vi "Demo_Main.vi"() -> ()   [LabVIEW 2016]
uses:
  ControlCAN/ControlCAN.llb/DevType.ctl
  ControlCAN/ControlCAN.llb/CAN Channel.ctl
  ControlCAN/ControlCAN.llb/InitFlag.ctl
  ControlCAN/ControlCAN.llb/Mode.ctl
  ControlCAN/ControlCAN.llb/Fliter.ctl
  ControlCAN/ControlCAN.llb/VCI_CAN_OBJ.ctl
  ControlCAN/ControlCAN.llb/VCI_INIT_CONFIG.ctl
  ControlCAN/ControlCAN.llb/Return Val.ctl
  ControlCAN/ControlCAN.lvlib
panel:
  in  "元素 8":u8 format="%x"
  in  "元素 7":u8 format="%x"
  in  "元素 6":u8 format="%x"
  in  "元素 5":u8 format="%x"
  in  "元素 4":u8 format="%x"
  in  "元素 3":u8 format="%x"
  in  "元素 2":u8 format="%x"
  in  "元素":u8 format="%x"
  in  "单选按钮 3":enum32{"未选择", "逆转", "顺转", "输出锁定"}(radio)=enum."输出锁定"
  in  "ID_VCU_MCU_1 2":u32=150013185 format="0x%x"
  out "vcu1 2":u32[](array[numeric]) format="%x"
  out "vcu1":u32[](array[numeric]) format="%x"
  out "vcu2":u32[](array[numeric]) format="%x"
  out "控制器温度":i16
  in  "list":i32(listbox)
  out "vcu3":u32[](array[numeric]) format="%x"
  in  "Data":string="01 00"
  in  "Format":u8(ring)=1 items=["标准帧", "扩展帧"]
  in  "Type":u8(ring) items=["数据帧", "远程帧"]
  in  "ID":u32 format="0x%x"
  in  "Send":bool
  out "Open":bool
  in  "Open 2":bool
  in  "Close":bool
  in  "kBaudRate":u8(ring)=10 caption="波特率" items=["5k bps"=1, "10k bps"=2, "20k bps"=3, "40k bps"=4, "50k bps"=5, "80k bps"=6, "100k bps"=7, "125k bps"=8, "200k bps"=9, "250k bps"=10, "400k bps"=11, "500k bps"=12, "666k bps"=13, "800k bps"=14, "1000k bps"=15, "33.33k bps"=16, "66.66k bps"=17, "83.33k bps"=18]
  in  "Channel":T1 caption="CAN通道" items=["通道1", "通道2"]
  in  "DevType":T2=3 caption="设备类型" items=["USB-CAN"=2, "USB-CAN2"=3]
  in  "RcvEnable":bool=TRUE
  in  "InitFlag":T3=1 caption="初始化参数" items=["使用Flash参数", "使用界面设置参数"]
  out "选项卡控件":enum32{"VCU控制", "CAN基本操作"}(tab)
  in  "驱动/制动":enum32{"未选择", "N", "L"}(radio)=enum."N"
  in  "车辆动力":enum32{"未选择", "N", "L", "R"}(radio)=enum."R"
  in  "车辆状态":enum32{"未选择", "N", "L", "R"}(radio)=enum."L"
  in  "充电状态":T4(radio)=enum."单选选项1 4"
  in  "状态信息1":T4(radio)=enum."空"
  in  "ID_VCU_MCU_2 2":u32=150078721 format="0x%x"
  in  "ID_VCU_MCU_1":u32=150013185 format="0x%x"
  in  "单选按钮":enum32{"未选择", "运行", "停止"}(radio)=enum."停止"
  in  "单选按钮 2":enum32{"未选择", "牵引", "制动"}(radio)=enum."制动"
  in  "ID_VCU_MCU_33":u32=150930689 format="0x%x"
  in  "状态信息2":T5(radio)
  in  "报警信息":enum32{"未选择", "N", "L", "R", "R 2"}(radio)
  in  "制动":dbl(knob) scale=0.0..5.0
  in  "油门":dbl(knob) scale=0.0..5.0
  out "油门":dbl
  out "转矩":dbl
  out "转速":dbl
  out "单选按钮 4":enum32{"未选择", "逆转", "顺转", "输出锁定"}(radio)
  out "单选按钮 5":enum32{"未选择", "牵引", "制动"}(radio)
  out "单选按钮 6":enum32{"未选择", "运行", "停止"}(radio)
  out "布尔数组":bool[](array[boolean])
  out "母线电压":u16
  out "电机相电流":dbl
  out "电机实际功率":dbl
  out "电机温度":i16
  in  "Clear":bool
  in  "Mode":T6 caption="工作模式" items=["正常工作", "仅侦听模式", "自测模式（环回）"]
  in  "Fliter":T7=1 items=["接收所有类型"=1, "只接收标准帧"=2, "只接收扩展帧"=3]
  in  "AccMask":u32=4294967295 caption="接收屏蔽码" format="%08x"
  in  "AccCode":u32 caption="接收过滤码" format="%08x"
  out "SendCnt":u32 caption="发送统计"
  out "RecvCnt":u32 caption="接收统计"
  # "位置传感器故障"
  # "过流"
  # "控制器过温"
  # "电机过温"
  # "欠压报警"
  # "过压报警"
  # "通讯故障"
  # "控制器高温"
  # "短路保护"
  # "严重欠压"
  # "超过峰值功率"
  # "超过最高限速"
  # "VCU故障"
  # "跛行状态"
  # "堵转保护"
  # "致命故障"
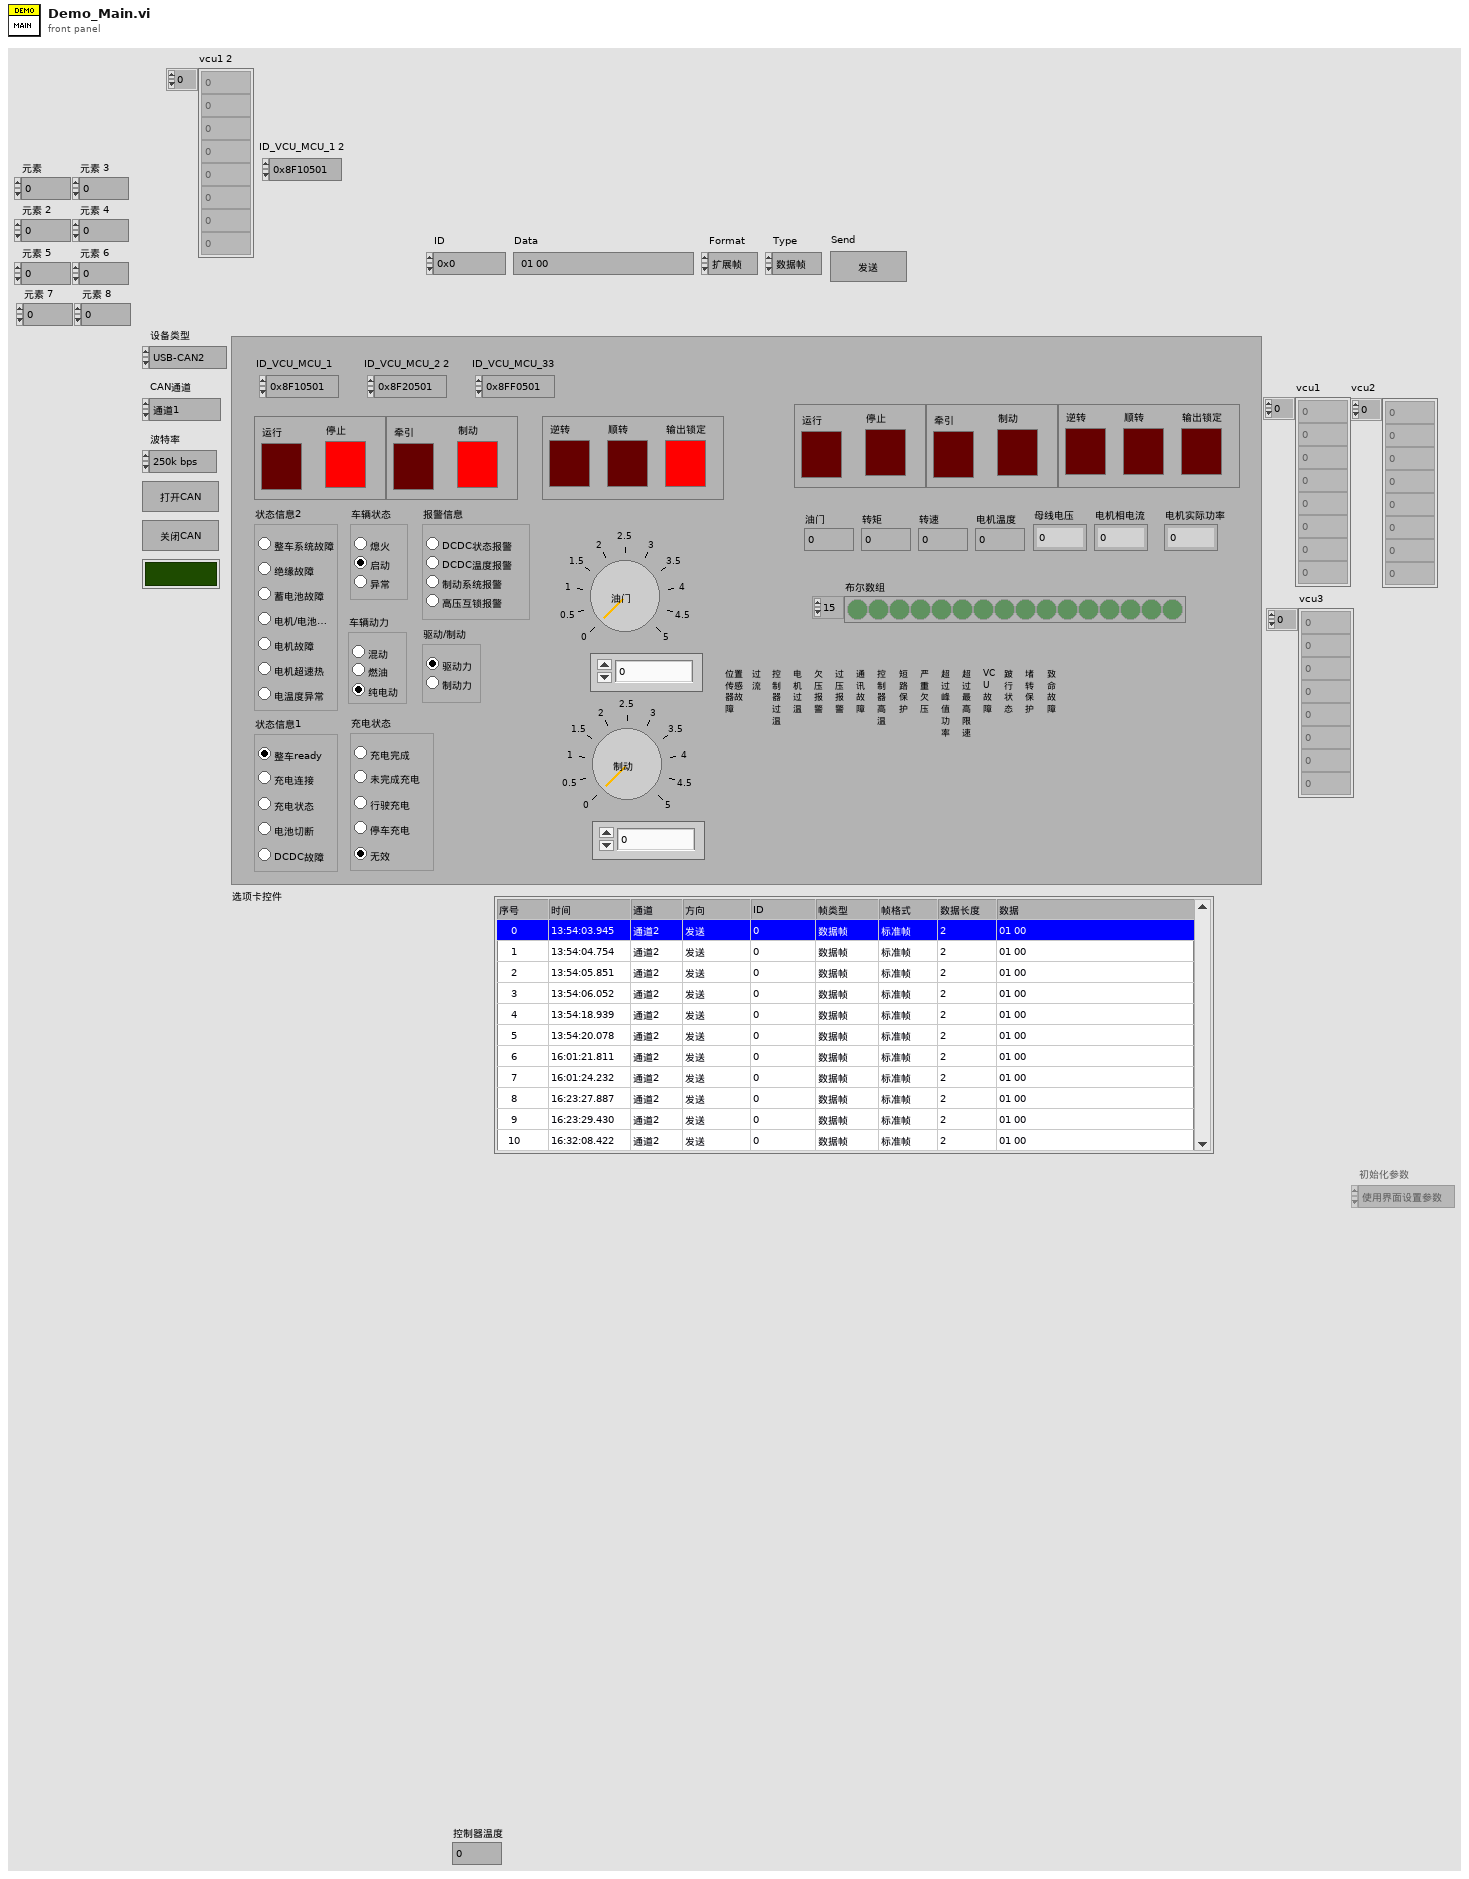
[diagram p1: front panel]
types:
  T1 = typedef "ControlCAN.lvlib/CAN Channel.ctl" = u32
  T2 = typedef "ControlCAN.lvlib/DevType.ctl" = u32
  T3 = typedef "ControlCAN.lvlib/InitFlag.ctl" = u32
  T4 = enum32{"未选择", "空", "速度控制", "转矩控制", "主动放电", "单选选项1 4"}
  T5 = enum32{"未选择", "空", "速度控制", "转矩控制", "主动放电", "单选选项1 4", "主动放电 2", "单选选项1 5"}
  T6 = typedef "ControlCAN.lvlib/Mode.ctl" = u8
  T7 = typedef "ControlCAN.lvlib/Fliter.ctl" = u8
  T8 = typedef "ControlCAN.lvlib/VCI_CAN_OBJ.ctl" = cluster{"ID":u32, "TimeStamp":u32, "TimeFlag":u8, "SendType":u8, "RemoteFlag":u8, "ExternFlag":u8, "DataLen":u8, "Data":u8[], "Reserved":u8[]}
  T9 = cluster{"Type":enum16{"接收", "发送"}, "Channel":T1, "Time":timestamp, "VCI_CAN_OBJ":T8}[]
  T10 = cluster{"Type":enum16{"接收", "发送"}, "Channel":T1, "Time":timestamp, "VCI_CAN_OBJ":T8}
  T11 = typedef "ControlCAN.lvlib/VCI_INIT_CONFIG.ctl" = cluster{"AccCode":u32, "AccMask":u32, "InitFlag":T3, "Fliter":T7, "Timing0":u8, "Timing1":u8, "Mode":T6}
  T12 = cluster{"DevType":T2, "DevIndex":u32, "CanIndex":T1, "VCI_INIT_CONFIG":T11}
  T13 = typedef "ControlCAN.lvlib/Return Val.ctl" = i32
  T14 = enum32{"invalid app kind", "Development System", "Run Time System", "Student Edition", "Embedded LabVIEW", "Evaluation", "Custom"}
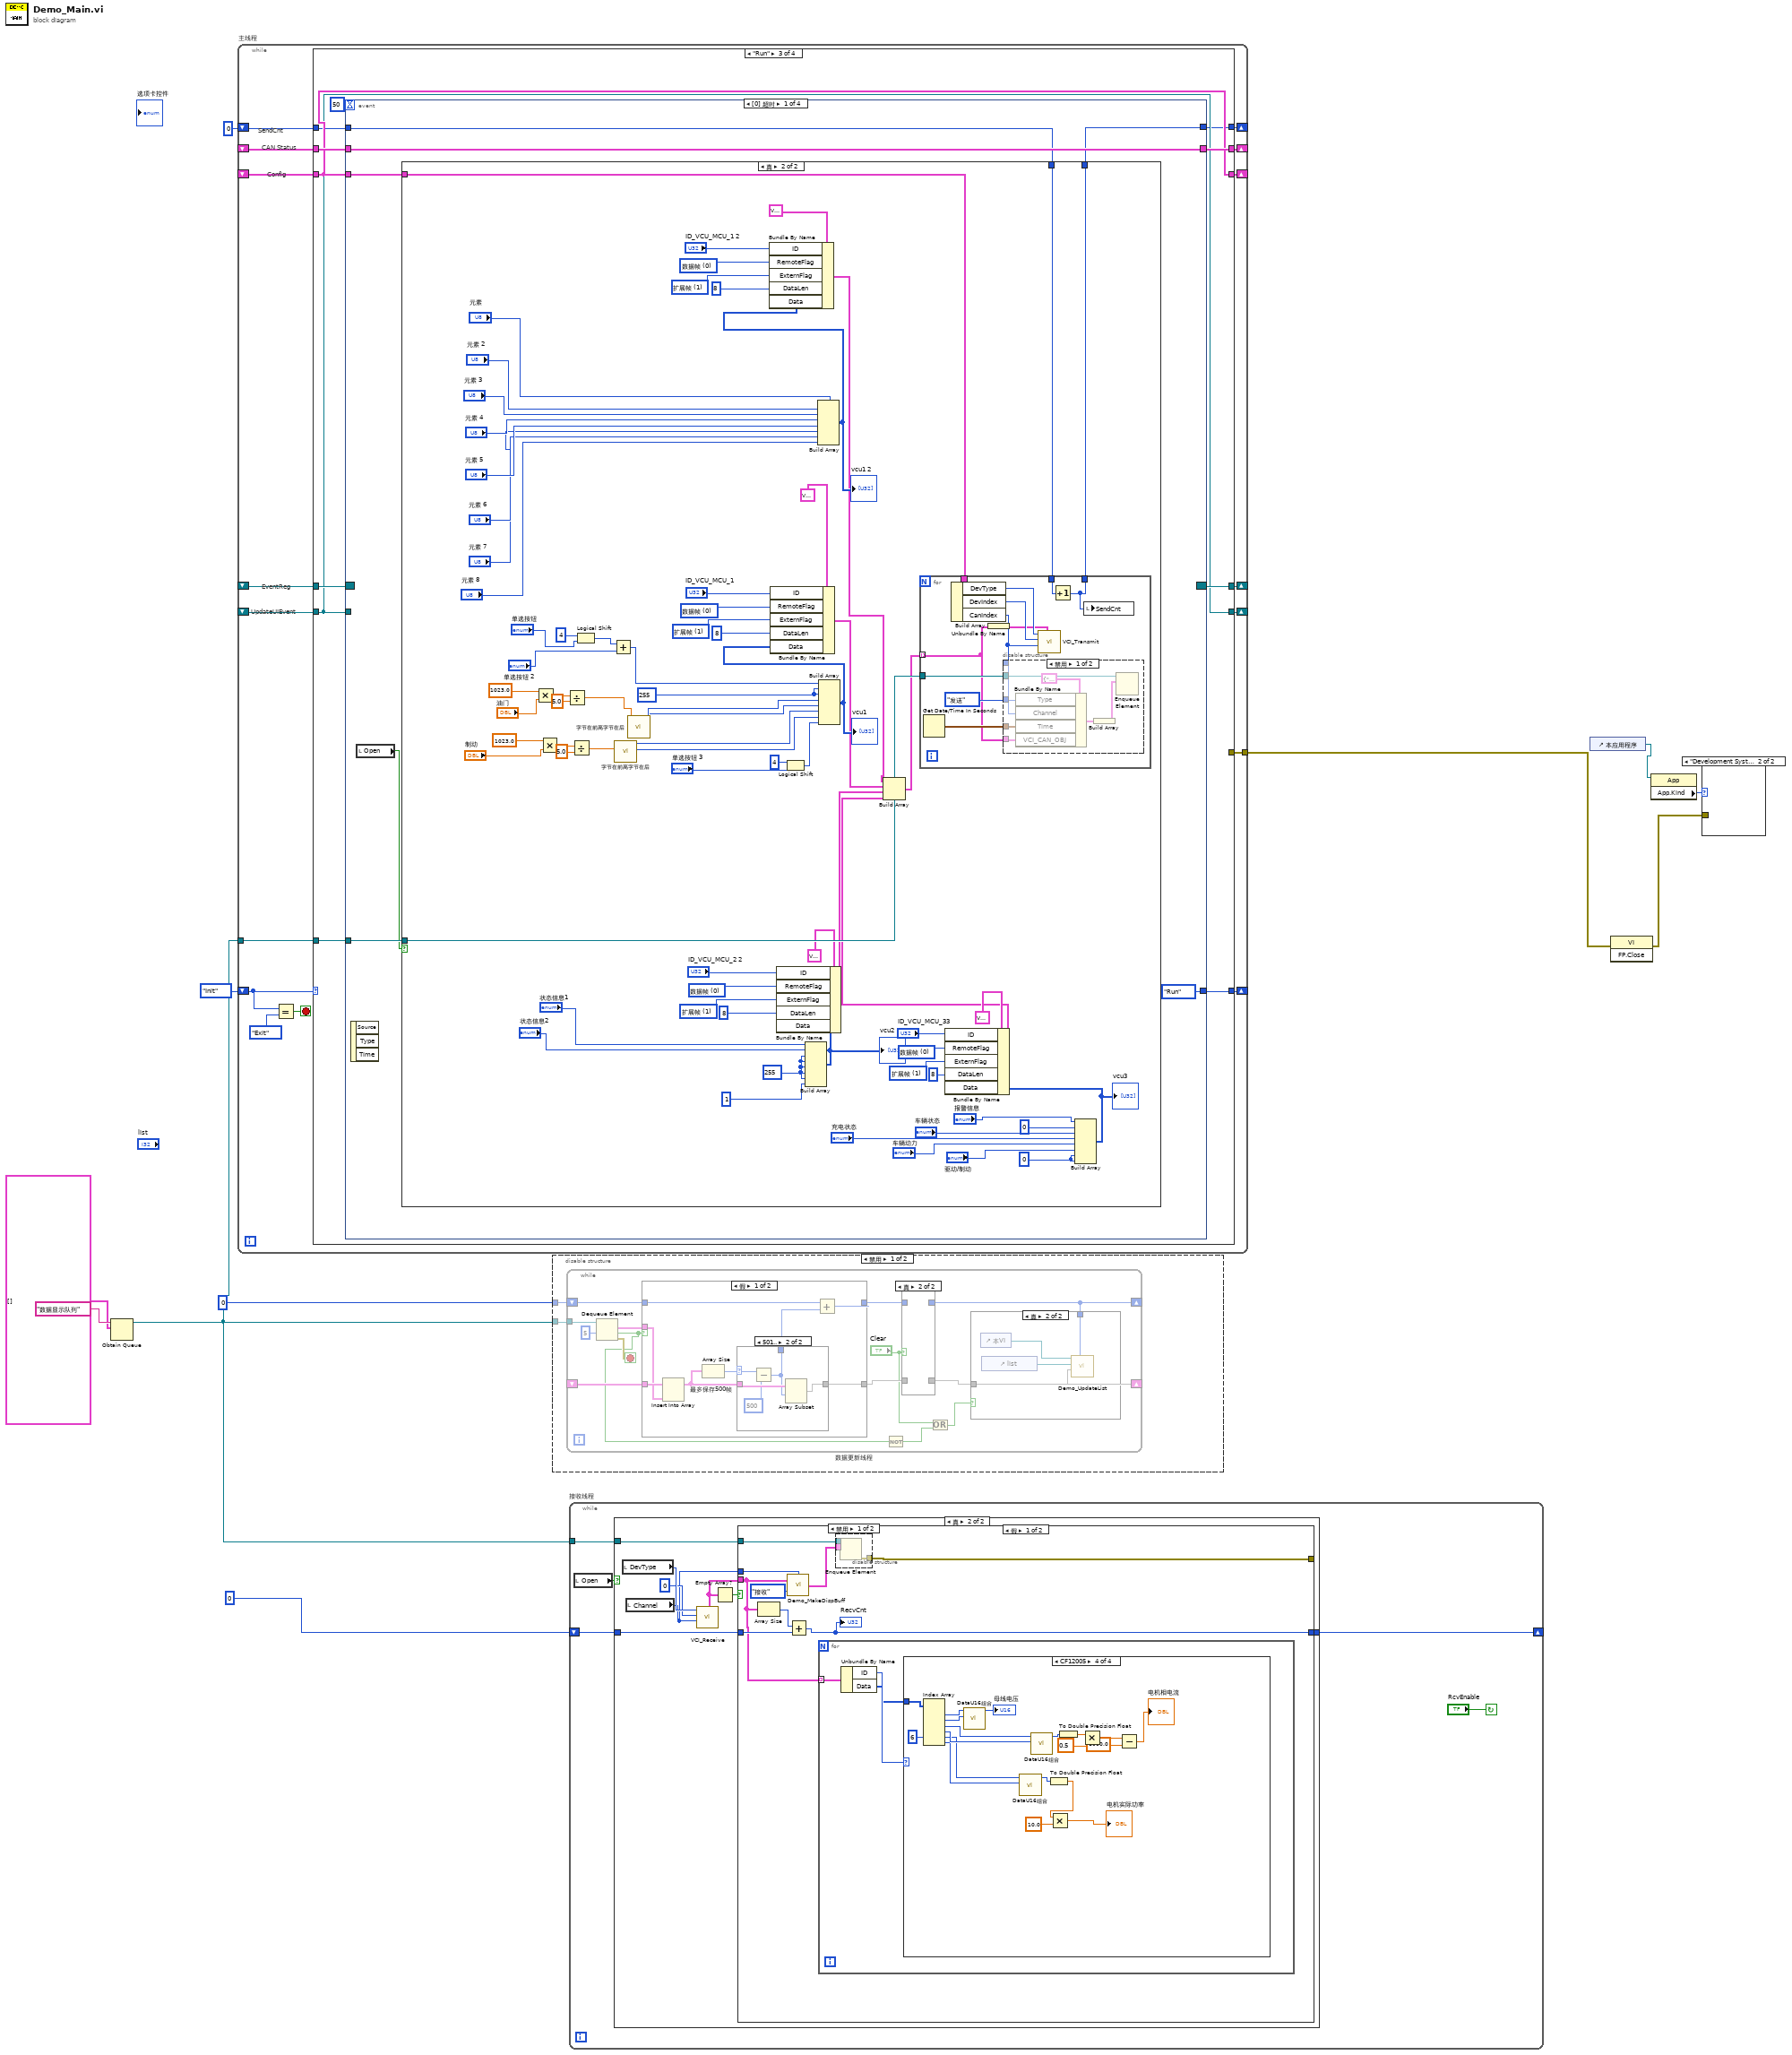
[diagram p0: block diagram]
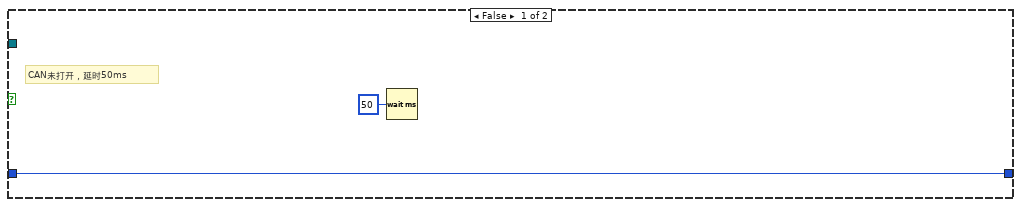
[diagram p7: hidden frame]
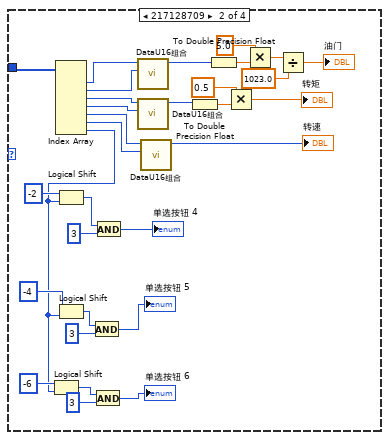
[diagram p10: hidden frame]
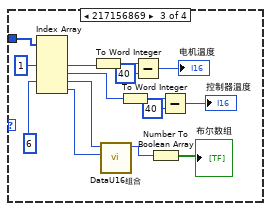
[diagram p11: hidden frame]
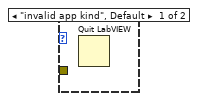
[diagram p13: hidden frame]
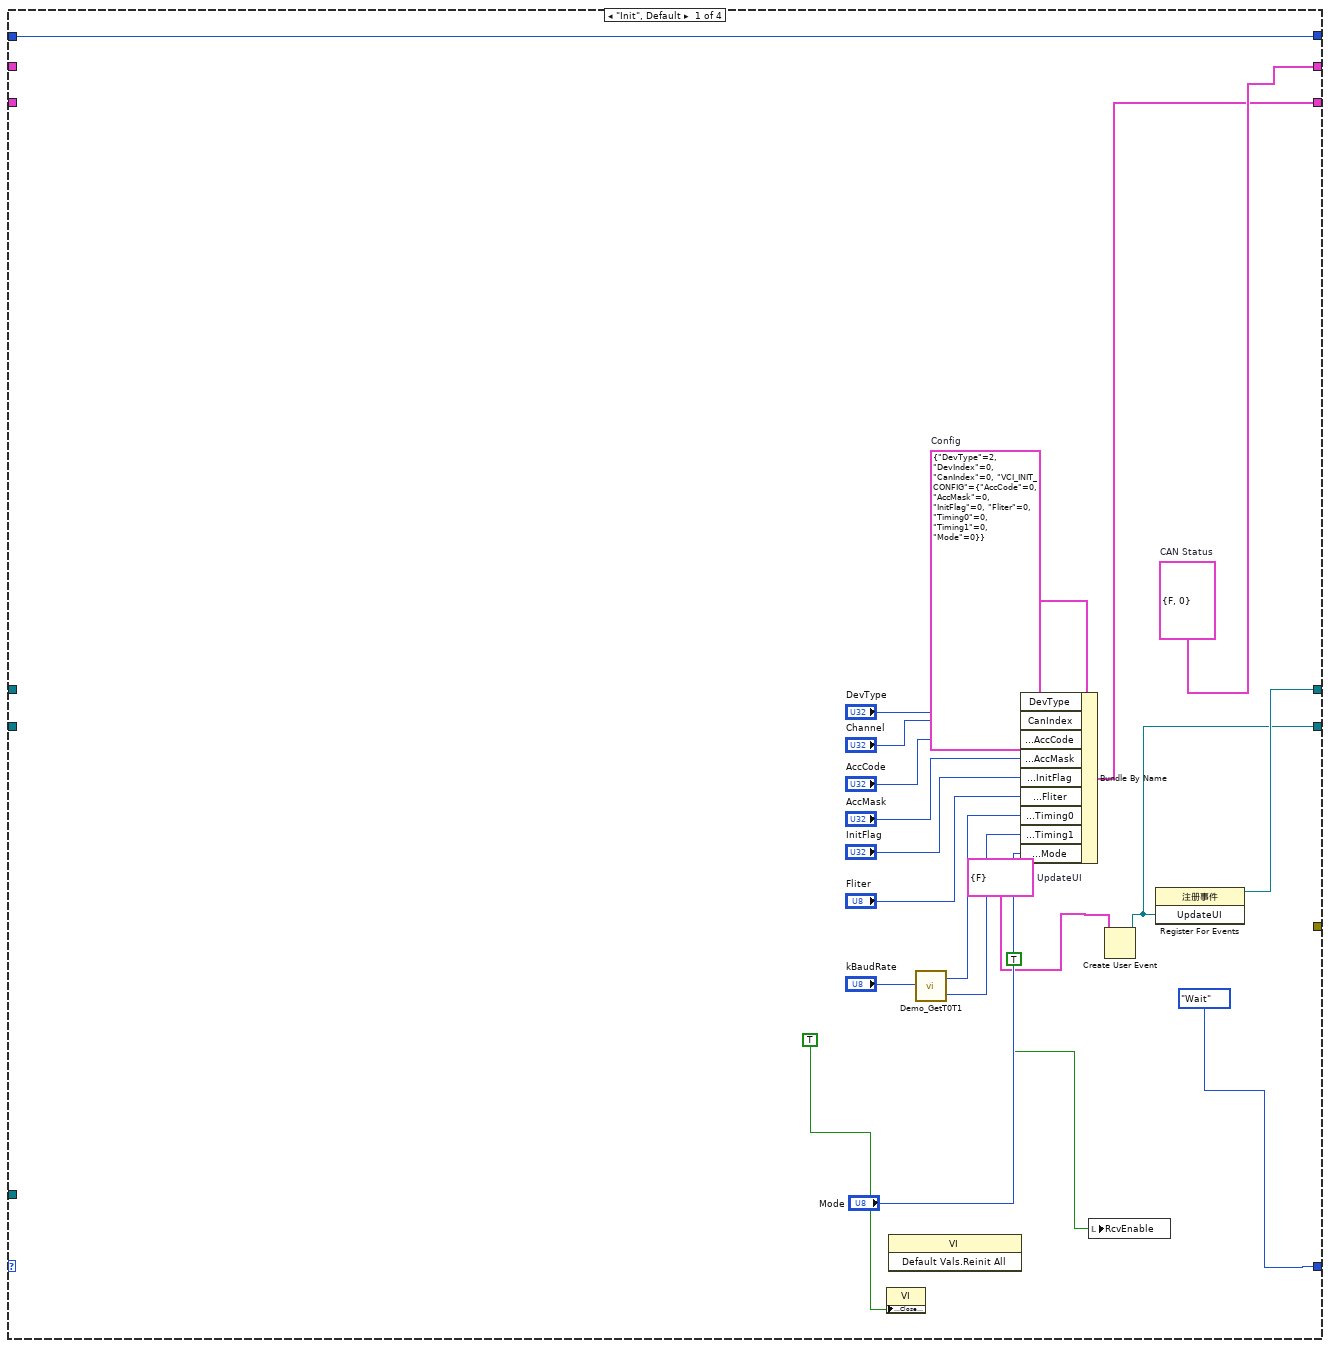
[diagram p14: hidden frame]
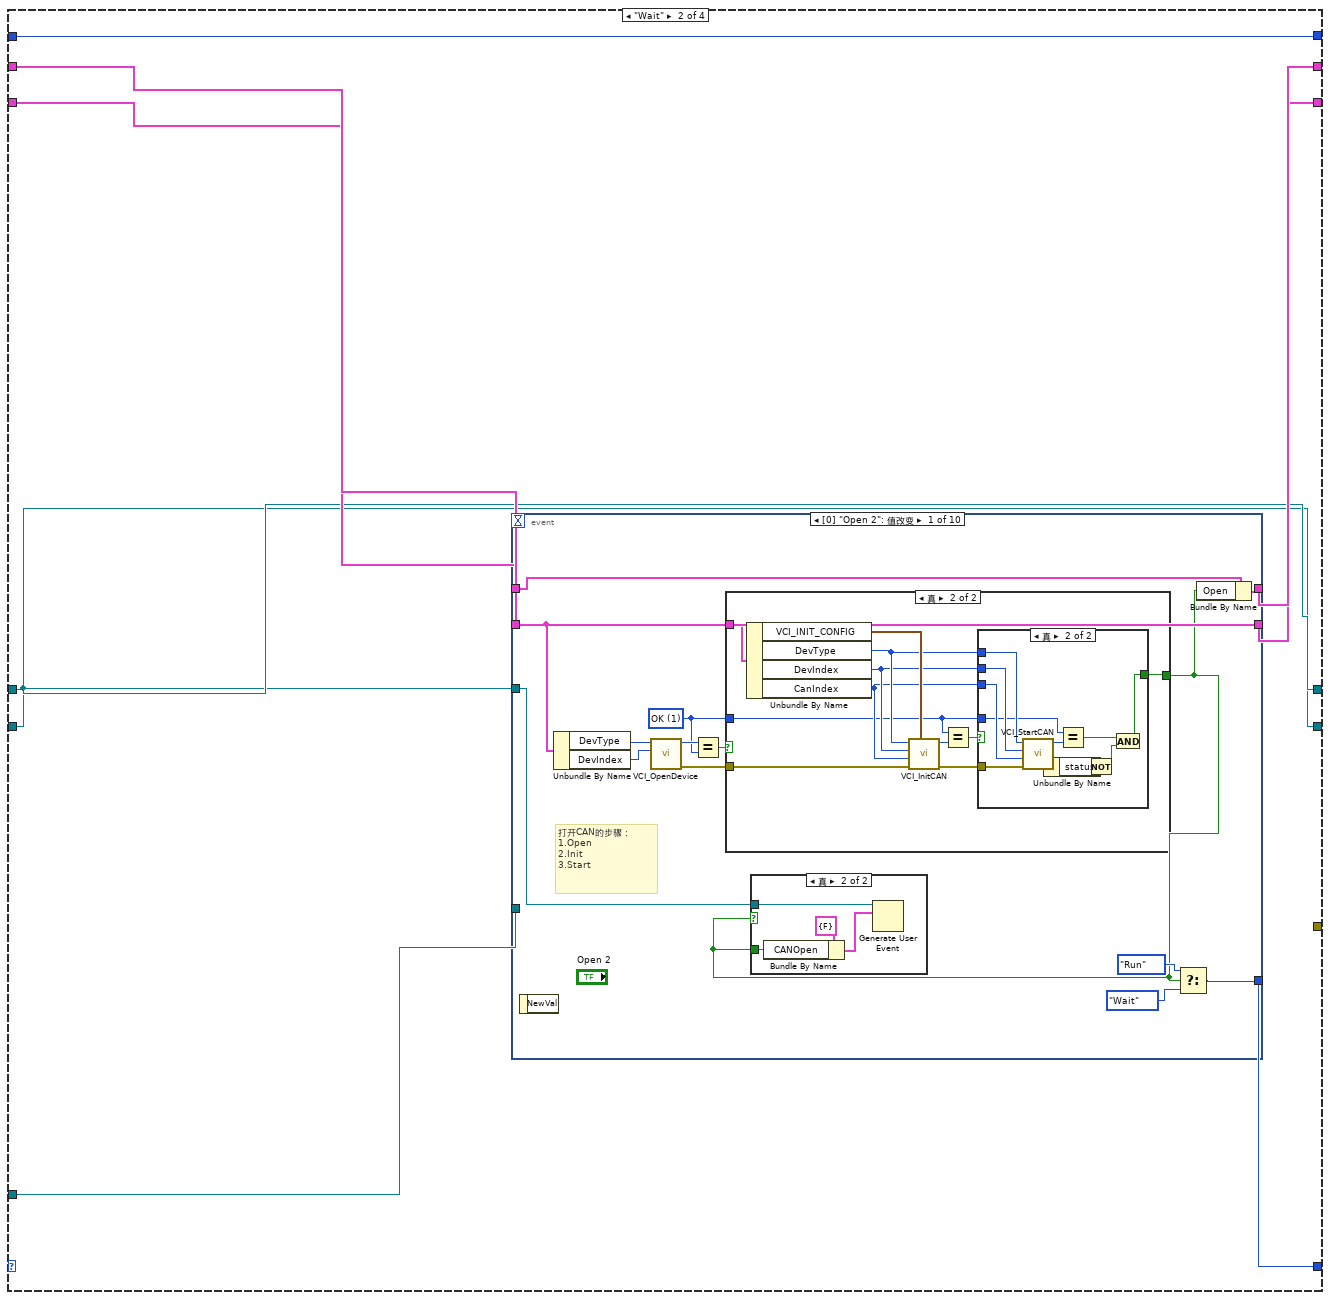
[diagram p15: hidden frame]
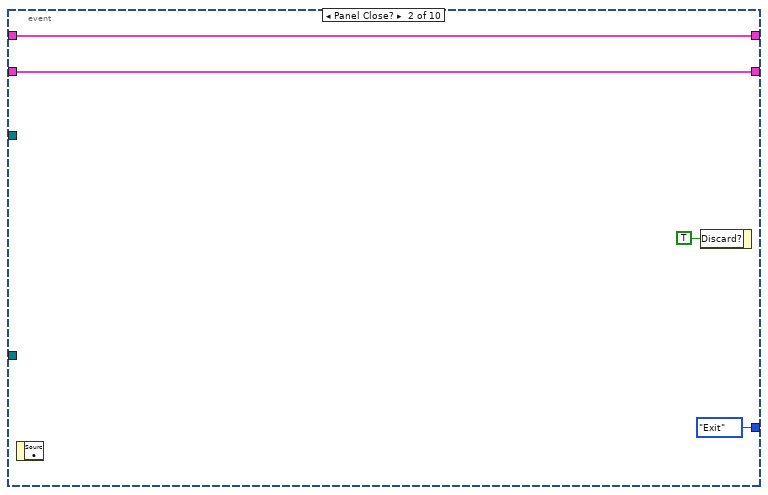
[diagram p19: hidden frame]
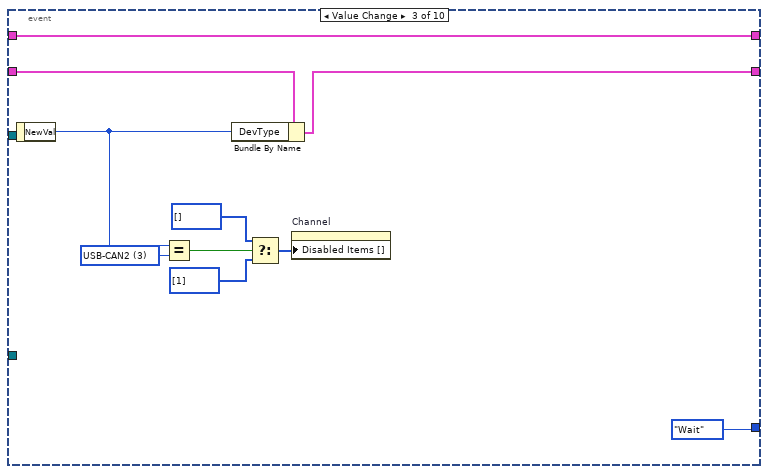
[diagram p20: hidden frame]
diagram:
  n1 = Obtain Queue(name (unnamed)="数据显示队列" ("名称（未命名）"), element data type=T9 []) -> (queue out=w8:refnum<queue>)  [unwired: 3 in, 2 out]
  n2 = while "主线程" {
    shift-right: [w23] -> _
    shift-left: enum16{"Init", "Wait", "Run", "Exit"}."Init" -> [w26]
    shift-right: [w24] -> _
    shift-left: _ -> [w25]
    shift-right: [w22] -> _
    shift-left: _ -> [w21]
    tunnel: w8 -> [w20]
    shift-right: [w18] -> _
    shift-left: _ -> [w17]
    shift-right: [w16] -> _
    shift-left: _ -> [w15]
    shift-right: [w13] -> _
    shift-left: u32 0 -> [w14]
    tunnel: [w12] -> w2
    stop <- w27 stop-if-true
    # "CAN Status"
    # "Config"
    # "EventReg"
    # "UpdateUIEvent"
    # "SendCnt"
    n3 = Equal?(x=w26, y=enum16{"Init", "Wait", "Run", "Exit"}."Exit") -> (x = y?=w27:bool)
    n4 = case shown="\"Run\"" w26 {
      tunnel: w25 -> [_ w56 w156 w316]
      tunnel: [w47 w55 w155 w316] -> w24
      tunnel: [enum16{"Init", "Wait", "Run", "Exit"}."Wait" w52 w158 enum16{"Init", "Wait", "Run", "Exit"}."Exit"] -> w23
      tunnel: [w43 w53 w154 w314] -> w22
      tunnel: w21 -> [_ w54 w154 w314]
      tunnel: w20 -> [_ w51 w157 w320]
      tunnel: [w35 w50 w152 w319] -> w18
      tunnel: w17 -> [_ w50 w153 w319]
      tunnel: [w34 w49 w151 w317] -> w16
      tunnel: w15 -> [_ w49 w151 w317]
      tunnel: w14 -> [w32 w48 w150 w312]
      tunnel: [w32 w48 w149 w312] -> w13
      tunnel: [_ _ _ errorcluster {"status"=FALSE, "code"=0, "source"=""} ("error constant")] -> w12
      frame "Init", Default {
        w36 = cluster{"CANOpen":bool} {"CANOpen"=FALSE}  # UpdateUI
        w46 = T12 {"DevType"=2, "DevIndex"=0, "CanIndex"=0, "VCI_INIT_CONFIG"={"AccCode"=0, "AccMask"=0, "InitFlag"=0, "Fliter"=0, "Timing0"=0, "Timing1"=0, "Mode"=0}}  # Config
        w47 = cluster{"Open":bool, "SendCnt":u32} {"Open"=FALSE, "SendCnt"=0}  # CAN Status
        n5 = property class="VI"("Front Panel.Closeable"=TRUE ("前面板窗口:可关闭")) -> ()  [unwired: 2 in, 2 out]
        n6 = invoke class="VI" method="Default Vals.Reinit All"() -> ()  [unwired: 3 in, 3 out]
        n7 = call "Demo_GetT0T1.vi"("kBaudRate"="kBaudRate") -> ("Timing0"=w29:u8, "Timing1"=w28:u8)
        n8 = Bundle By Name(cluster=w46, "DevType"="DevType", "CanIndex"="Channel", "VCI_INIT_CONFIG.AccCode"="AccCode", "VCI_INIT_CONFIG.AccMask"="AccMask", "VCI_INIT_CONFIG.InitFlag"="InitFlag", "VCI_INIT_CONFIG.Fliter"="Fliter", "VCI_INIT_CONFIG.Timing0"=w29, "VCI_INIT_CONFIG.Timing1"=w28, "VCI_INIT_CONFIG.Mode"="Mode") -> (w43:T12)
        n9 = local write "RcvEnable"(TRUE ("RcvEnable")) -> ()
        n10 = Create User Event(user event datatype=w36) -> (user event=w34:refnum<user-event>)  [unwired: 1 in, 1 out]
        n11 = register-events(w34) -> (reference out=w35:refnum<event-registration>)  [unwired: 2 in, 1 out]
      }
      frame "Wait" {
        n12 = event shown="[0] \"Open 2\": 值改变" {
          selector: _ -> [_ _ _ _ _ _ _ _ _ _]
          dyn-events: _ -> [_ _ _ _ _ _ _ _ _ _]
          timeout: _ -> [_ _ _ _ _ _ _ _ _ _]
          tunnel: w56 -> [w60 w100 w110 w115 w120 w125 w130 w135 w142 w147]
          tunnel: [w59 w100 w110 w115 w120 w125 w130 w135 w142 w147] -> w55
          tunnel: w54 -> [w70 w99 w109 w114 w119 w124 w129 w134 w141 w146]
          tunnel: [w70 w99 w108 w112 w117 w122 w127 w132 w140 w144] -> w53
          tunnel: [w61 enum16{"Init", "Wait", "Run", "Exit"}."Exit" enum16{"Init", "Wait", "Run", "Exit"}."Wait" enum16{"Init", "Wait", "Run", "Exit"}."Wait" enum16{"Init", "Wait", "Run", "Exit"}."Wait" enum16{"Init", "Wait", "Run", "Exit"}."Wait" enum16{"Init", "Wait", "Run", "Exit"}."Wait" enum16{"Init", "Wait", "Run", "Exit"}."Wait" enum16{"Init", "Wait", "Run", "Exit"}."Wait" enum16{"Init", "Wait", "Run", "Exit"}."Wait"] -> w52
          tunnel: w51 -> [_ _ _ _ _ _ _ _ _ _]
          tunnel: w49 -> [w58 _ _ _ _ _ _ _ _ _]
          event "Open 2": Value Change {
            w64 = T13 1 items=["OK"=1, "ERROR1"=0, "ERROR2"=-1] ("y")
            # "打开CAN的步骤：\n1.Open\n2.Init\n3.Start"
            n13 = event-data() -> ()  [unwired: 2 out]
            n14 = Unbundle By Name(w70) -> ("DevType"=w69:T2, "DevIndex"=w68:u32)
            n15 = call "VCI_OpenDevice.vi"("DevIndex"=w68, "DevType"=w69) -> ("error out"=w65:errorcluster, "Return Val"=w67:T13)  [unwired: 2 in, 6 out]
            n16 = Equal?(x=w67, y=w64) -> (x = y?=w66:bool)
            n17 = case shown="真" w66 {
              tunnel: w65 -> [_ w85]
              tunnel: w70 -> [_ w84]
              tunnel: w64 -> [_ w76]
              tunnel: [_ w75] -> w57
              frame False {
              }
              frame True {
                n18 = Unbundle By Name(w84) -> ("VCI_INIT_CONFIG"=w83:T11, "DevType"=w79:T2, "DevIndex"=w78:u32, "CanIndex"=w77:T1)
                n19 = call "VCI_InitCAN.vi"("VCI_INIT_CONFIG"=w83, "error in (no error)"=w85, "CANIndex"=w77, "DevIndex"=w78, "DevType"=w79) -> ("error out"=w80:errorcluster, "Return Val"=w82:T13)  [unwired: 5 out]
                n20 = Equal?(x=w76, y=w82) -> (x = y?=w81:bool)
                n21 = case shown="真" w81 {
                  tunnel: w80 -> [_ w96]
                  tunnel: w79 -> [_ w95]
                  tunnel: w78 -> [_ w94]
                  tunnel: w77 -> [_ w93]
                  tunnel: w76 -> [_ w91]
                  tunnel: [_ w87] -> w75
                  frame False {
                  }
                  frame True {
                    n22 = call "VCI_StartCAN.vi"("error in (no error)"=w96, "CANIndex"=w93, "DevIndex"=w94, "DevType"=w95) -> ("error out"=w89:errorcluster, "Return Val"=w92:T13)  [unwired: 6 out]
                    n23 = Unbundle By Name(w89) -> ("status"=w86:bool)
                    n24 = Equal?(x=w91, y=w92) -> (x = y?=w90:bool)
                    n25 = Not(x=w86) -> (.not. x?=w88:bool)
                    n26 = And(x=w90, y=w88) -> (x .and. y?=w87:bool)
                  }
                }
              }
            }
            n27 = case shown="真" w57 {
              tunnel: w58 -> [_ w74]
              tunnel: w57 -> [_ w72]
              frame False {
              }
              frame True {
                n28 = Bundle By Name(cluster=cluster{"CANOpen":bool} {"CANOpen"=FALSE} ("事件数据"), "CANOpen"=w72) -> (w71:cluster{"CANOpen":bool})
                n29 = Generate User Event(user event=w74, event data cluster=w71) -> ()  [unwired: 2 in, 2 out]
              }
            }
            n30 = Select(t=enum16{"Init", "Wait", "Run", "Exit"}."Run", s=w57, f=enum16{"Init", "Wait", "Run", "Exit"}."Wait") -> (s? t:f=w61:enum16{"Init", "Wait", "Run", "Exit"})
            n31 = Bundle By Name(cluster=w60, "Open"=w57) -> (w59:cluster{"Open":bool, "SendCnt":u32})
          }
          event Panel Close? {
            n32 = event-data() -> ()  [unwired: 2 out]
            n33 = event-data("Discard?"=TRUE ("放弃？")) -> ()  [unwired: 1 in, 1 out]
          }
          event Value Change {
            w106 = T2 3 items=["USB-CAN"=2, "USB-CAN2"=3] ("y")
            n34 = event-data() -> ("NewVal"=w107:T2)  [unwired: 1 out]
            n35 = Equal?(x=w107, y=w106) -> (x = y?=w105:bool)
            n36 = Bundle By Name(cluster=w109, "DevType"=w107) -> (w108:T12)
            n37 = Select(t=i32[] [] ("禁用项[]"), s=w105, f=i32[] [1] ("禁用项[]")) -> (s? t:f=w104:i32[])
            n38 = property on="Channel" class="Ring (严格)"("Disabled Items []"=w104) -> ()  [unwired: 2 in, 2 out]
          }
          event Value Change {
            n39 = event-data() -> ("NewVal"=w113:T1)  [unwired: 1 out]
            n40 = Bundle By Name(cluster=w114, "CanIndex"=w113) -> (w112:T12)
          }
          event "AccCode": Value Change {
            n41 = event-data() -> ("NewVal"=w118:u32)  [unwired: 1 out]
            n42 = Bundle By Name(cluster=w119, "VCI_INIT_CONFIG.AccCode"=w118) -> (w117:T12)
          }
          event "AccMask": Value Change {
            n43 = event-data() -> ("NewVal"=w123:u32)  [unwired: 1 out]
            n44 = Bundle By Name(cluster=w124, "VCI_INIT_CONFIG.AccMask"=w123) -> (w122:T12)
          }
          event Value Change {
            n45 = event-data() -> ("NewVal"=w128:T3)  [unwired: 1 out]
            n46 = Bundle By Name(cluster=w129, "VCI_INIT_CONFIG.InitFlag"=w128) -> (w127:T12)
          }
          event Value Change {
            n47 = event-data() -> ("NewVal"=w133:T6)  [unwired: 1 out]
            n48 = Bundle By Name(cluster=w134, "VCI_INIT_CONFIG.Mode"=w133) -> (w132:T12)
          }
          event "kBaudRate": Value Change {
            n49 = event-data() -> ("NewVal"=w138:u8)  [unwired: 1 out]
            n50 = call "Demo_GetT0T1.vi"("kBaudRate"=w138) -> ("Timing0"=w137:u8, "Timing1"=w136:u8)
            n51 = Bundle By Name(cluster=w141, "VCI_INIT_CONFIG.Timing0"=w137, "VCI_INIT_CONFIG.Timing1"=w136) -> (w140:T12)
          }
          event Value Change {
            n52 = event-data() -> ("NewVal"=w145:T7)  [unwired: 1 out]
            n53 = Bundle By Name(cluster=w146, "VCI_INIT_CONFIG.Fliter"=w145) -> (w144:T12)
          }
        }
      }
      frame "Run" {
        n54 = event shown="[0] 超时" {
          selector: w153 -> [_ _ _ _]
          dyn-events: [_ _ _ _] -> w152
          timeout: 50 -> [_ _ _ _]
          tunnel: [enum16{"Init", "Wait", "Run", "Exit"}."Run" enum16{"Init", "Wait", "Run", "Exit"}."Run" enum16{"Init", "Wait", "Run", "Exit"}."Run" w307] -> w158
          tunnel: w157 -> [w162 w271 _ _]
          tunnel: [w164 w282 w289 w308] -> w155
          tunnel: w156 -> [w164 w282 w291 w308]
          tunnel: w154 -> [w163 w277 w296 _]
          tunnel: w151 -> [_ _ w288 _]
          tunnel: w150 -> [w160 w266 w284 w306]
          tunnel: [w161 w265 w284 w306] -> w149
          event Timeout {
            n55 = event-data() -> ()  [unwired: 4 out]
            n56 = local read "Open"() -> (w159:bool)
            n57 = case shown="真" w159 {
              tunnel: w163 -> [_ w238]
              tunnel: w162 -> [_ w237]
              tunnel: [w166 w224] -> w161
              tunnel: w160 -> [w166 w223]
              frame False {
              }
              frame True {
                w178 = u8 1 items=["标准帧", "扩展帧"] ("Format 2")
                w177 = u8 0 items=["数据帧", "远程帧"] ("Type 2")
                w183 = u8 0 ("元素")
                w190 = u8 255
                w205 = u8 255
                w216 = u8 1 items=["标准帧", "扩展帧"] ("Format 2")
                w217 = u8 0 items=["数据帧", "远程帧"] ("Type 2")
                w230 = u8 1 items=["标准帧", "扩展帧"] ("Format 2")
                w229 = u8 0 items=["数据帧", "远程帧"] ("Type 2")
                w239 = u8 1 items=["标准帧", "扩展帧"] ("Format 2")
                w240 = u8 0 items=["数据帧", "远程帧"] ("Type 2")
                n58 = Multiply(x=1023.0, y="油门") -> (x*y=w204:dbl)
                n59 = Multiply(x=1023.0, y="制动") -> (x*y=w199:dbl)
                n60 = Divide(x=w204, y=5.0) -> (x/y=w202:dbl)
                n61 = Divide(x=w199, y=5.0) -> (x/y=w201:dbl)
                n62 = Logical Shift(y=i16 4, x="单选按钮") -> (x << y=w209:u32)
                n63 = Add(x=w209, y="单选按钮 2") -> (x+y=w206:u32)
                n64 = call "字节在前高字节在后.vi"("数值输入"=w201) -> ("高字节"=w195:u16, "低字节"=w196:u8)  [unwired: 9 in]
                n65 = call "字节在前高字节在后.vi"("数值输入"=w202) -> ("高字节"=w219:u16, "低字节"=w220:u8)  [unwired: 9 in]
                n66 = Logical Shift(y=i16 4, x="单选按钮 3") -> (x << y=w193:u32)
                n67 = Build Array("状态信息1", "状态信息2", w190, w190, w190, w190, w190, u8 1) -> (w233:u32[])
                "vcu2" <- w233
                n68 = Bundle By Name(cluster=T8 {"ID"=0, "TimeStamp"=0, "TimeFlag"=0, "SendType"=0, "RemoteFlag"=0, "ExternFlag"=0, "DataLen"=0, "Data"=[], "Reserved"=[]} ("Send"), "ID"="ID_VCU_MCU_2 2", "RemoteFlag"=w229, "ExternFlag"=w230, "DataLen"=u8 8, "Data"=w233) -> (w227:T8)
                n69 = Build Array("元素", "元素 2", "元素 3", "元素 4", "元素 5", "元素 6", "元素 7", "元素 8") -> (w181:u8[])
                "vcu1 2" <- w181
                n70 = Bundle By Name(cluster=T8 {"ID"=0, "TimeStamp"=0, "TimeFlag"=0, "SendType"=0, "RemoteFlag"=0, "ExternFlag"=0, "DataLen"=0, "Data"=[], "Reserved"=[]} ("Send"), "ID"="ID_VCU_MCU_1 2", "RemoteFlag"=w177, "ExternFlag"=w178, "DataLen"=u8 8, "Data"=w181) -> (w175:T8)
                n71 = Build Array(w206, w205, w205, w220, w219, w196, w195, w193) -> (w234:u32[])
                "vcu1" <- w234
                n72 = Bundle By Name(cluster=T8 {"ID"=0, "TimeStamp"=0, "TimeFlag"=0, "SendType"=0, "RemoteFlag"=0, "ExternFlag"=0, "DataLen"=0, "Data"=[], "Reserved"=[]} ("Send"), "ID"="ID_VCU_MCU_1", "RemoteFlag"=w240, "ExternFlag"=w239, "DataLen"=u8 8, "Data"=w234) -> (w226:T8)
                n73 = Build Array("报警信息", u8 0 ("元素"), "车辆状态", "充电状态", "车辆动力", "驱动/制动", w183, w183) -> (w211:u32[])
                "vcu3" <- w211
                n74 = Bundle By Name(cluster=T8 {"ID"=0, "TimeStamp"=0, "TimeFlag"=0, "SendType"=0, "RemoteFlag"=0, "ExternFlag"=0, "DataLen"=0, "Data"=[], "Reserved"=[]} ("Send"), "ID"="ID_VCU_MCU_33", "RemoteFlag"=w217, "ExternFlag"=w216, "DataLen"=u8 8, "Data"=w211) -> (w212:T8)
                n75 = Build Array(w175, w226, w227, w212) -> (w225:T8[])
                n76 = for {
                  tunnel: w238 -> [w252]
                  tunnel: w237 -> [w249]
                  tunnel: w225 -> [w244] mode=indexing
                  tunnel: w223 -> [w243]
                  tunnel: [w242] -> w224
                  n77 = Get Date/Time In Seconds() -> (seconds since 1Jan1904=w246:timestamp)
                  n78 = Unbundle By Name(w252) -> ("DevType"=w251:T2, "DevIndex"=w250:u32, "CanIndex"=w247:T1)
                  n79 = Build Array(w244) -> (w245:T8[])
                  n80 = disable-structure shown="禁用" {
                    disable-tunnel: w249 -> [w260 _]
                    disable-tunnel: enum16{"接收", "发送"}."发送" ("Type") -> [w258 _]
                    disable-tunnel: w247 -> [w257 _]
                    disable-tunnel: w246 -> [w256 _]
                    disable-tunnel: w244 -> [w253 _]
                    frame Disabled {
                      n81 = Bundle By Name(cluster=T10 {"Type"=enum."发送", "Channel"=0, "Time"=timestamp(0 s since 1904-01-01), "VCI_CAN_OBJ"={"ID"=0, "TimeStamp"=0, "TimeFlag"=0, "SendType"=0, "RemoteFlag"=0, "ExternFlag"=0, "DataLen"=0, "Data"=[], "Reserved"=[]}}, "Type"=w258, "Channel"=w257, "Time"=w256, "VCI_CAN_OBJ"=w253) -> (w255:T10)
                      n82 = Build Array(w255) -> (w254:T9)
                      n83 = Enqueue Element(queue=w260, element=w254) -> ()  [unwired: 1 in, 4 out]
                    }
                    frame Enabled {
                    }
                  }
                  n84 = call "VCI_Transmit.vi"("Buffer"=w245, "CANIndex"=w247, "DevIndex"=w250, "DevType"=w251) -> ()  [unwired: 1 in, 7 out]
                  n85 = Increment(x=w243) -> (x+1=w242:u32)
                  n86 = local write "SendCnt"(w242) -> ()
                }
              }
            }
          }
          event "Send": Value Change {
            n87 = event-data() -> ()  [unwired: 2 out]
            n88 = Increment(x=w266) -> (x+1=w265:u32)
            "SendCnt" <- w265
            n89 = call "Demo_MakeData.vi"("DataString"="Data") -> ("Data"=w272:u8[], "DataLen"=w273:u8)  [unwired: 9 out]
            n90 = Bundle By Name(cluster=T8 {"ID"=0, "TimeStamp"=0, "TimeFlag"=0, "SendType"=0, "RemoteFlag"=0, "ExternFlag"=0, "DataLen"=0, "Data"=[], "Reserved"=[]} ("Send"), "ID"="ID", "RemoteFlag"="Type", "ExternFlag"="Format", "DataLen"=w273, "Data"=w272) -> (w263:T8)
            n91 = Build Array(w263) -> (w264:T8[])
            n92 = Get Date/Time In Seconds() -> (seconds since 1Jan1904=w267:timestamp)
            n93 = Unbundle By Name(w277) -> ("DevType"=w276:T2, "DevIndex"=w275:u32, "CanIndex"=w268:T1)
            n94 = Bundle By Name(cluster=T10 {"Type"=enum."发送", "Channel"=0, "Time"=timestamp(0 s since 1904-01-01), "VCI_CAN_OBJ"={"ID"=0, "TimeStamp"=0, "TimeFlag"=0, "SendType"=0, "RemoteFlag"=0, "ExternFlag"=0, "DataLen"=0, "Data"=[], "Reserved"=[]}}, "Type"=enum16{"接收", "发送"}."发送", "Channel"=w268, "Time"=w267, "VCI_CAN_OBJ"=w263) -> (w262:T10)
            n95 = call "VCI_Transmit.vi"("Buffer"=w264, "CANIndex"=w268, "DevIndex"=w275, "DevType"=w276) -> ()  [unwired: 1 in, 7 out]
            n96 = Build Array(w262) -> (w261:T9)
            n97 = Enqueue Element(queue=w271, element=w261) -> ()  [unwired: 1 in, 4 out]
          }
          event "Close": Value Change {
            w292 = T13 1 items=["OK"=1, "ERROR1"=0, "ERROR2"=-1] ("y")
            n98 = event-data() -> ()  [unwired: 2 out]
            n99 = Unbundle By Name(w296) -> ("DevType"=w295:T2, "DevIndex"=w294:u32)
            n100 = call "VCI_CloseDevice.vi"("DevIndex"=w294, "DevType"=w295) -> ("Return Val"=w293:T13)  [unwired: 1 in, 8 out]
            n101 = Equal?(x=w293, y=w292) -> (x = y?=w290:bool)
            n102 = Not(x=w290) -> (.not. x?=w286:bool)
            n103 = Bundle By Name(cluster=cluster{"CANOpen":bool} {"CANOpen"=FALSE} ("事件数据"), "CANOpen"=w286) -> (w285:cluster{"CANOpen":bool})
            n104 = Bundle By Name(cluster=w291, "Open"=w286) -> (w289:cluster{"Open":bool, "SendCnt":u32})
            n105 = local write "Open"(w286) -> ()
            n106 = Generate User Event(user event=w288, event data cluster=w285) -> ()  [unwired: 2 in, 2 out]
          }
          event User Event {
            w303 = 0
            w302 = 2
            n107 = event-data() -> ("CANOpen"=w305:bool)  [unwired: 1 out]
            "Open" <- w305
            n108 = Not(x=w305) -> (.not. x?=w298:bool)
            n109 = Select(t=w302, s=w305, f=w303) -> (s? t:f=w304:i32)
            n110 = Select(t=w303, s=w305, f=w302) -> (s? t:f=w299:i32)
            n111 = property class="VI"("Front Panel.Closeable"=w298) -> ()  [unwired: 2 in, 2 out]
            n112 = Select(t=enum16{"Init", "Wait", "Run", "Exit"}."Run", s=w305, f=enum16{"Init", "Wait", "Run", "Exit"}."Wait") -> (s? t:f=w307:enum16{"Init", "Wait", "Run", "Exit"})
            n113 = disable-structure shown="禁用" {
              disable-tunnel: w304 -> [w310 _]
              disable-tunnel: w299 -> [w309 _]
              frame Disabled {
                n114 = property on="Close" class="Bool"("DisabledEnum"=w309) -> ()  [unwired: 2 in, 2 out]
                n115 = property on="ID" class="DigNum (严格)"("DisabledEnum"=w309) -> ()  [unwired: 2 in, 2 out]
                n116 = property on="Data" class="Str"("DisabledEnum"=w309) -> ()  [unwired: 2 in, 2 out]
                n117 = property on="Format" class="Ring (严格)"("DisabledEnum"=w309) -> ()  [unwired: 2 in, 2 out]
                n118 = property on="Type" class="Ring (严格)"("DisabledEnum"=w309) -> ()  [unwired: 2 in, 2 out]
                n119 = property on="Send" class="Bool"("DisabledEnum"=w309) -> ()  [unwired: 2 in, 2 out]
                n120 = property on="Clear" class="Bool"("DisabledEnum"=w309) -> ()  [unwired: 2 in, 2 out]
                n121 = property on="Fliter" class="Ring (严格)"("DisabledEnum"=w310) -> ()  [unwired: 2 in, 2 out]
                n122 = property on="DevType" class="Ring (严格)"("DisabledEnum"=w310) -> ()  [unwired: 2 in, 2 out]
                n123 = property on="Channel" class="Ring (严格)"("DisabledEnum"=w310) -> ()  [unwired: 2 in, 2 out]
                n124 = property on="AccCode" class="DigNum (严格)"("DisabledEnum"=w310) -> ()  [unwired: 2 in, 2 out]
                n125 = property on="AccMask" class="DigNum (严格)"("DisabledEnum"=w310) -> ()  [unwired: 2 in, 2 out]
                n126 = property on="InitFlag" class="Ring (严格)"("DisabledEnum"=w310) -> ()  [unwired: 2 in, 2 out]
                n127 = property on="Mode" class="Ring (严格)"("DisabledEnum"=w310) -> ()  [unwired: 2 in, 2 out]
                n128 = property on="kBaudRate" class="Ring (严格)"("DisabledEnum"=w310) -> ()  [unwired: 2 in, 2 out]
                n129 = property on="Open 2" class="Bool"("DisabledEnum"=w310) -> ()  [unwired: 2 in, 2 out]
              }
              frame Enabled {
              }
            }
          }
        }
      }
      frame "Exit" {
        n130 = Release Queue(queue=w320) -> ()  [unwired: 1 in, 4 out]
        n131 = Unregister For Events(event registration refnum=w319) -> (error out=w318:errorcluster)  [unwired: 1 in]
        n132 = Destroy User Event(user event=w317, error in=w318) -> ()  [unwired: 1 out]
        n133 = Unbundle By Name(w316) -> ("Open"=w315:bool)
        n134 = local write "RcvEnable"(FALSE ("RcvEnable")) -> ()
        n135 = case shown="真" w315 {
          tunnel: w314 -> [_ w324]
          frame False {
          }
          frame True {
            n136 = Unbundle By Name(w324) -> ("DevType"=w323:T2, "DevIndex"=w322:u32)
            n137 = call "VCI_CloseDevice.vi"("DevIndex"=w322, "DevType"=w323) -> ()  [unwired: 1 in, 9 out]
          }
        }
      }
    }
  }
  n138 = disable-structure shown="禁用" {
    disable-tunnel: w8 -> [w326 _]
    disable-tunnel: 0 -> [w325 _]
    frame Disabled {
      n139 = while "数据更新线程" {
        tunnel: w326 -> [w340]
        shift-right: [w331] -> _
        shift-left: _ -> [w336]
        shift-right: [w332] -> _
        shift-left: w325 -> [w335]
        stop <- w338 stop-if-true
        n140 = Dequeue Element(queue=w340, timeout in ms (-1)=5 ("超时毫秒(-1)")) -> (element=w337:T9, timed out?=w330:bool, error out=w338:errorcluster)  [unwired: 1 in, 1 out]
        n141 = case shown="假" w330 {
          tunnel: w337 -> [w351 _]
          tunnel: w336 -> [w354 w362]
          tunnel: [w347 w362] -> w334
          tunnel: w335 -> [w350 w361]
          tunnel: [w348 w361] -> w333
          frame False {
            n142 = Insert Into Array(array=w354, new element=w351) -> (w352:T9)  [unwired: 1 in]
            n143 = Array Size(array=w352) -> (size(s)=w353:i32)
            n144 = case "最多保存500帧" shown="501.." w353 {
              selector: w353 -> [_ w359]
              tunnel: w352 -> [w355 w360]
              tunnel: [w355 w357] -> w347
              tunnel: [_ w356] -> w349
              frame 0, Default {
              }
              frame 501.. {
                n145 = Subtract(x=w359, y=500) -> (x-y=w356:i32)
                n146 = Array Subset(array=w360, index=w356) -> (w357:T9)  [unwired: 1 in]
              }
            }
            n147 = Add(x=w350, y=w349) -> (x+y=w348:i32)
          }
          frame True {
          }
        }
        n148 = Not(x=w330) -> (.not. x?=w329:bool)
        n149 = case shown="真" "Clear" {
          tunnel: w333 -> [w345 _]
          tunnel: w334 -> [w346 _]
          tunnel: [w346 _] -> w331
          tunnel: [w345 _] -> w332
          frame False {
          }
          frame True {
          }
        }
        n150 = Or(x="Clear", y=w329) -> (x .or. y?=w328:bool)
        n151 = case shown="真" w328 {
          tunnel: w332 -> [_ w342]
          tunnel: w331 -> [_ w341]
          frame False {
          }
          frame True {
            n152 = control-ref of="本VI"() -> (w343:refnum<vi>)
            n153 = control-ref of="list"() -> (w344:refnum<vi>)
            n154 = call "Demo_UpdateList.vi"("Offset"=w342, "Buffer"=w341, "list"=w344, "MainVi"=w343) -> ()  [unwired: 8 out]
          }
        }
      }
    }
    frame Enabled {
    }
  }
  n155 = while "接收线程" {
    tunnel: w8 -> [w365]
    shift-right: [w363] -> _
    shift-left: u32 0 ("RecvCnt") -> [w364]
    stop <- "RcvEnable" continue-if-true
    n156 = local read "Open"() -> (w366:bool)
    n157 = case shown="真" w366 {
      tunnel: w365 -> [_ w373]
      tunnel: w364 -> [w368 w372]
      tunnel: [w368 w371] -> w363
      frame False {
        # "CAN未打开，延时50ms"
        n158 = Wait (ms)(milliseconds to wait=u32 50 ("等待时间（毫秒）")) -> ()  [unwired: 1 out]
      }
      frame True {
        n159 = local read "DevType"() -> (w377:T2)
        n160 = local read "Channel"() -> (w370:T1)
        n161 = call "VCI_Receive.vi"("CANIndex"=w370, "DevIndex"=u32 0, "DevType"=w377) -> ("Recieve"=w374:T8[])  [unwired: 3 in, 5 out]
        n162 = Empty Array?(array=w374) -> (empty?=w375:bool)
        n163 = case shown="假" w375 {
          tunnel: w373 -> [w386 _]
          tunnel: w374 -> [w378 _]
          tunnel: [w383 _] -> _
          tunnel: w372 -> [w381 w458]
          tunnel: [w380 w458] -> w371
          tunnel: w370 -> [w379 _]
          frame False {
            n164 = Array Size(array=w378) -> (size(s)=w382:i32)
            n165 = call "Demo_MakeDispBuff.vi"("Channel"=w379, "Type"=enum16{"接收", "发送"}."接收", "OBJs"=w378) -> ("Buffer"=w384:T9)
            n166 = Add(x=w382, y=w381) -> (x+y=w380:u32)
            "RecvCnt" <- w380
            n167 = for {
              tunnel: w378 -> [w392] mode=indexing
              n168 = Unbundle By Name(w392) -> ("ID"=w391:u32, "Data"=w390:u8[])
              n169 = case shown="CF12005" w391 {
                tunnel: w390 -> [_ w423 w438 w457]
                frame 0, Default {
                }
                frame 217128709 {
                  n170 = Index Array(array=w423) -> (element #1=w422:u8, element #2=w421:u8, element #3=w414:u8, element #4=w413:u8, element #5=w408:u8, element #6=w407:u8, element #7=w393:u8)  [unwired: 7 in]
                  n171 = Logical Shift(y=i16 -6, x=w393) -> (x << y=w397:u8)
                  n172 = Logical Shift(y=i16 -2, x=w393) -> (x << y=w401:u8)
                  n173 = Logical Shift(y=i16 -4, x=w393) -> (x << y=w399:u8)
                  n174 = And(x=w399, y=u8 3) -> (x .and. y?=→"单选按钮 5":u8)
                  n175 = And(x=w397, y=u8 3) -> (x .and. y?=→"单选按钮 6":u8)
                  n176 = And(x=w401, y=u8 3) -> (x .and. y?=→"单选按钮 4":u8)
                  n177 = call "DataU16组合.vi"("高字节"=w421, "低字节"=w422) -> ("数值输出"=w420:u16)  [unwired: 9 in]
                  n178 = call "DataU16组合.vi"("高字节"=w413, "低字节"=w414) -> ("数值输出"=w410:u16)  [unwired: 9 in]
                  n179 = call "DataU16组合.vi"("高字节"=w407, "低字节"=w408) -> ("数值输出"=→"转速":u16)  [unwired: 9 in]
                  n180 = To Double Precision Float(number=w410) -> (double precision float=w412:dbl)
                  n181 = To Double Precision Float(number=w420) -> (double precision float=w419:dbl)
                  n182 = Multiply(x=0.5, y=w412) -> (x*y=→"转矩":dbl)
                  n183 = Multiply(x=5.0, y=w419) -> (x*y=w417:dbl)
                  n184 = Divide(x=w417, y=1023.0) -> (x/y=→"油门":dbl)
                }
                frame 217156869 {
                  n185 = Index Array(array=w438, index #2=1 ("索引"), index #4=6 ("索引")) -> (element #2=w437:u8, element #3=w430:u8, element #4=w427:u8, element #5=w426:u8)  [unwired: 3 in, 1 out]
                  n186 = To Word Integer(number=w437) -> (16bit integer=w436:i16)
                  n187 = call "DataU16组合.vi"("高字节"=w426, "低字节"=w427) -> ("数值输出"=w425:u16)  [unwired: 9 in]
                  n188 = To Word Integer(number=w430) -> (16bit integer=w433:i16)
                  n189 = Subtract(x=w436, y=i16 40) -> (x-y=→"电机温度":i16)
                  n190 = Number To Boolean Array(number=w425) -> (Boolean array=→"布尔数组":bool[])
                  n191 = Subtract(x=w433, y=i16 40) -> (x-y=→"控制器温度":i16)
                }
                frame 217128965 {
                  n192 = Index Array(array=w457, index #5=6 ("索引")) -> (element #1=w456:u8, element #2=w455:u8, element #3=w453:u8, element #4=w452:u8, element #5=w450:u8, element #6=w449:u8)  [unwired: 5 in]
                  n193 = call "DataU16组合.vi"("高字节"=w455, "低字节"=w456) -> ("数值输出"=→"母线电压":u16)  [unwired: 9 in]
                  n194 = call "DataU16组合.vi"("高字节"=w449, "低字节"=w450) -> ("数值输出"=w448:u16)  [unwired: 9 in]
                  n195 = call "DataU16组合.vi"("高字节"=w452, "低字节"=w453) -> ("数值输出"=w444:u16)  [unwired: 9 in]
                  n196 = To Double Precision Float(number=w448) -> (double precision float=w447:dbl)
                  n197 = Multiply(x=w447, y=10.0) -> (x*y=→"电机实际功率":dbl)
                  n198 = To Double Precision Float(number=w444) -> (double precision float=w443:dbl)
                  n199 = Multiply(x=w443, y=0.5) -> (x*y=w441:dbl)
                  n200 = Subtract(x=w441, y=1000.0) -> (x-y=→"电机相电流":dbl)
                }
              }
            }
            n201 = disable-structure shown="禁用" {
              disable-tunnel: w386 -> [w389 _]
              disable-tunnel: w384 -> [w388 _]
              disable-tunnel: [w387 _] -> w383
              frame Disabled {
                n202 = Enqueue Element(queue=w389, element=w388) -> (error out=w387:errorcluster)  [unwired: 1 in, 3 out]
              }
              frame Enabled {
              }
            }
          }
          frame True {
          }
        }
      }
    }
  }
  n203 = control-ref of="本应用程序"() -> (w4:refnum<vi>)
  n204 = invoke class="VI" method="FP.Close"(error in=w2) -> (error out=w1:errorcluster)  [unwired: 2 in, 2 out]
  n205 = property class="App"(reference=w4) -> ("App.Kind"=w3:T14)  [unwired: 1 in, 2 out]
  n206 = case shown="\"Development System\"" w3 {
    tunnel: w1 -> [_ _]
    frame "invalid app kind", Default {
      n207 = Quit LabVIEW() -> ()  [unwired: 1 out]
    }
    frame "Development System" {
    }
  }
